vi "Teleop.vi"(10 "Match Info":T1={"Autonomous Elapsed Seconds"=0.0, "TeleOp Elapsed Seconds"=0.0, "Disabled Elapsed Seconds"=0.0, "Visited Autonomous"=FALSE, "Visited TeleOp"=FALSE, "Visited Disabled"=FALSE, "Autonomous Settings"={"Autonomous Style"=enum."Independent", "VI Refnum"=refnum}}, 11 "Call Context":T2) -> ()   [LabVIEW 2011]
doc: "This VI is called for each TeleOp packet received from the DS where the robot is not disabled. It is often used to read from the joysticks and update I/O or to update setpoints for timed control loops. It should complete and return within 20 milliseconds or it may miss DS packets."
uses:
  <vilib>/Rock Robotics/WPI/DriverStation/WPI_DriverStationDerivedRobotMode.ctl
  <vilib>/Rock Robotics/WPI/DriverStation/WPI_DriverStationMatch Info.ctl
  Robot Global Data.vi
panel:
  out "Position 4":dbl
  out "Position 3":dbl
  out "Shift Control":dbl=2.0 format="%.2f"
  in  "Left High":dbl=0.2
  in  "Right High":dbl=0.8
  in  "Left Mid":dbl=0.25
  in  "Right Mid":dbl=0.7
  in  "Shift Input 2":dbl
  in  "Left Low":dbl=0.8
  in  "Right Low":dbl=0.4
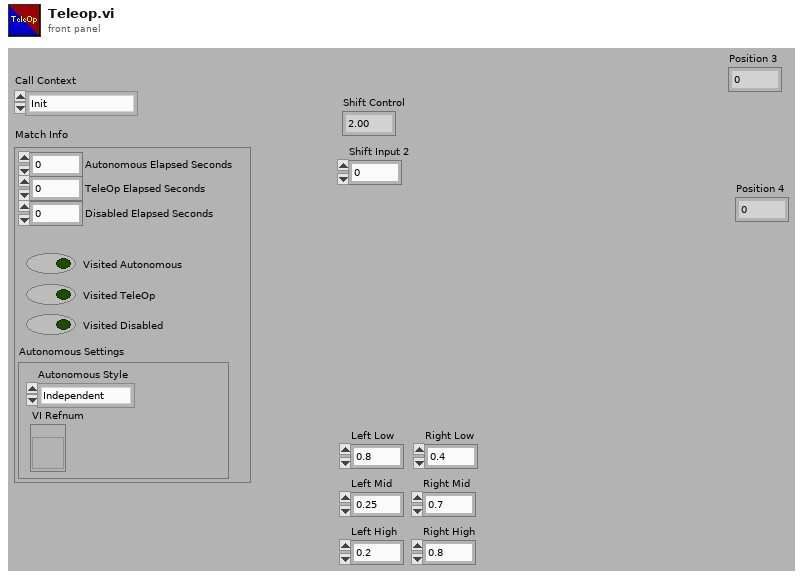
[diagram p1: front panel]
types:
  T1 = typedef "WPI_DriverStationMatch Info.ctl" = cluster{"Autonomous Elapsed Seconds":dbl, "TeleOp Elapsed Seconds":dbl, "Disabled Elapsed Seconds":dbl, "Visited Autonomous":bool, "Visited TeleOp":bool, "Visited Disabled":bool, "Autonomous Settings":cluster{"Autonomous Style":enum16{"Iterative", "Independent"}, "VI Refnum":refnum<vi>}}
  T2 = typedef "WPI_DriverStationDerivedRobotMode.ctl" = enum16{"Init", "Execute", "Stop"}
  T3 = typedef "WPI_JoystickDevRef.ctl" = cluster{"Device":T4}
  T4 = typedef "WPI_JoystickDeviceEnum.ctl" = enum16{"USB 1", "USB 2", "USB 3", "USB 4", "Kinect 1", "Kinect 2"}
  T5 = typedef "WPI_JoystickButtonState.ctl" = cluster{"Button 1":bool, "Button 2":bool, "Button 3":bool, "Button 4":bool, "Button 5":bool, "Button 6":bool, "Button 7":bool, "Button 8":bool, "Button 9":bool, "Button 10":bool, "Button 11":bool, "Button 12":bool}
  T6 = typedef "WPI_MotorControlDeviceRef.ctl" = cluster{"DeviceStatus":errorcluster, "Type":enum16{"PWM", "CAN"}, "PWM":cluster{"Digital Module":T7, "PWM Channel":T8, "DeadBand":T9}, "CAN":cluster{"Device Number":u8, "Control Mode":T10, "Semaphore":T11, "Max Vout":dbl}, "Invert":bool, "TransformRef":T12, "InvTransformRef":T12}
  T7 = typedef "FPGA_TypedefDigitalModule.ctl" = enum16{"Digital Module 1", "Digital Module 2"}
  T8 = typedef "FPGA_DIOPWMChannel.ctl" = enum8{"PWM 1", "PWM 2", "PWM 3", "PWM 4", "PWM 5", "PWM 6", "PWM 7", "PWM 8", "PWM 9", "PWM 10", "Invalid"}
  T9 = typedef "WPI_PWMDeadband.ctl" = cluster{"Name":string, "maxPositivePwm":i32, "minPositivePwm":i32, "centerPwm":i32, "maxNegativePwm":i32, "minNegativePwm":i32, "angularRange":u16}
  T10 = typedef "WPI_CANJaguar_ControlMode.ctl" = enum8{"Percent VBus", "Current", "Speed", "Position", "Voltage"}
  T11 = typedef "Semaphore RefNum" = refnum<k1>
  T12 = typedef "WPI_PWMTransform_ConPane.ctl" = refnum<vi>
  T13 = cluster{"axis 1 (x)":dbl, "axis 2 (y)":dbl, "axis 3 (throttle)":dbl, "axis 4":dbl, "axis 5":dbl, "axis 6":dbl}
  T14 = typedef "WPI_ServoDeviceRef.ctl" = cluster{"DeviceStatus":errorcluster, "Digital Module":T7, "PWM Channel":T8, "DeadBand":T9}
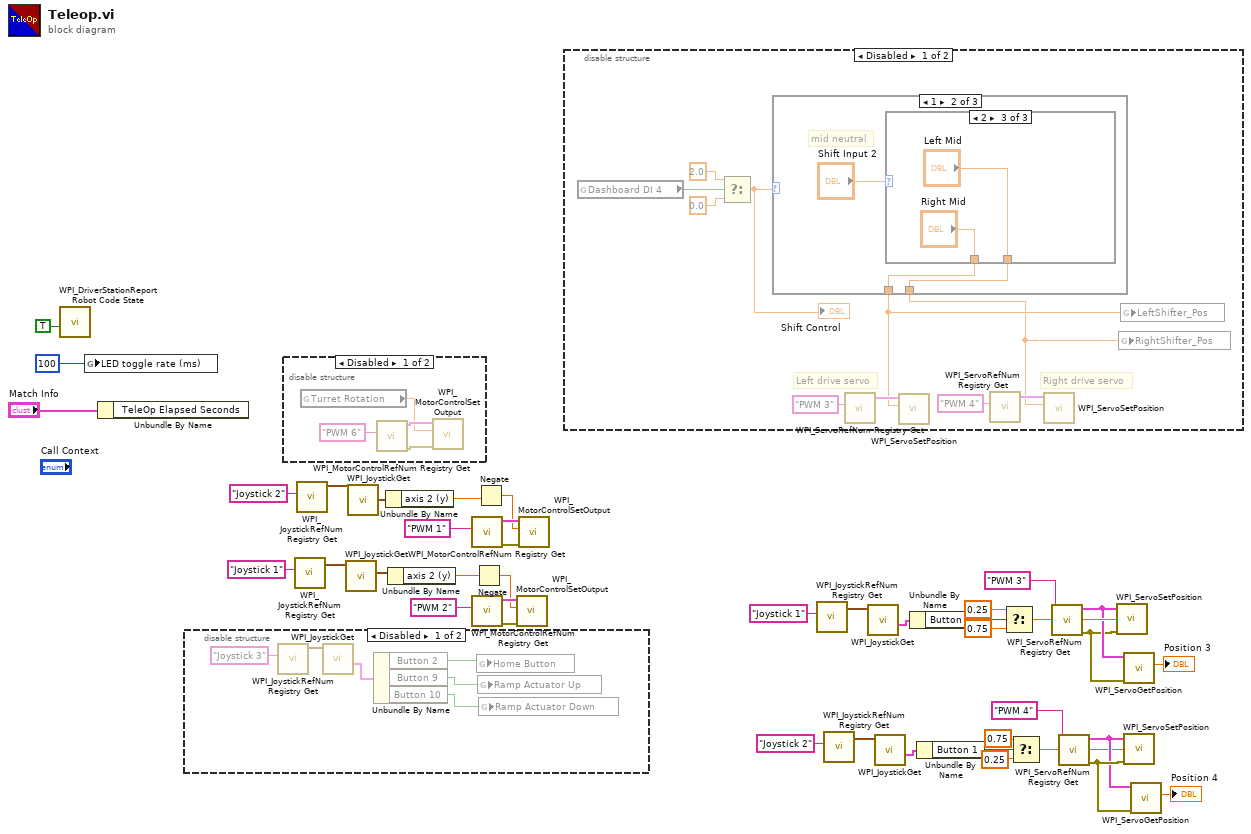
[diagram p0: block diagram]
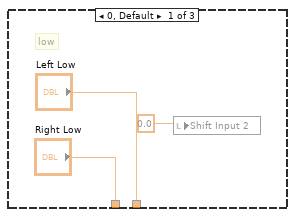
[diagram p4: hidden frame]
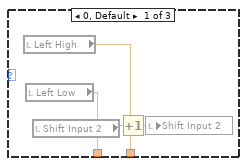
[diagram p5: hidden frame]
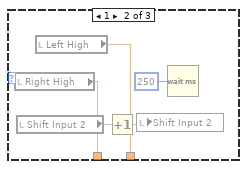
[diagram p6: hidden frame]
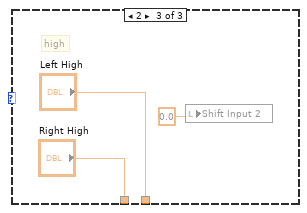
[diagram p7: hidden frame]
diagram:
  n1 = call <vilib>:"WPI_DriverStationReport Robot Code State.vi"("TeleOp"=TRUE ("Autonomous")) -> ()  [unwired: 10 in, 1 out]
  n2 = global write "Robot Global Data.vi" "LED toggle rate (ms)"(u32 100 ("LED ms toggle rate")) -> ()
  n3 = Unbundle By Name("Match Info") -> ()  [unwired: 1 out]
  n4 = disable-structure shown="Disabled" {
    frame Disabled {
      n5 = call <vilib>:"WPI_JoystickRefNum Registry Get.vi"("refnum name"="Joystick 3") -> ("JoystickDevRef"=w47:T3)  [unwired: 9 in, 1 out]
      n6 = call <vilib>:"WPI_JoystickGet.vi"("JoystickDevRef"=w47) -> ("Buttons"=w46:T5)  [unwired: 4 in, 2 out]
      n7 = Unbundle By Name(w46) -> ("Button 2"=w45:bool, "Button 9"=w43:bool, "Button 10"=w42:bool)
      n8 = global write "Robot Global Data.vi" "Home Button"(w45) -> ()
      n9 = global write "Robot Global Data.vi" "Ramp Actuator Up"(w43) -> ()
      n10 = global write "Robot Global Data.vi" "Ramp Actuator Down"(w42) -> ()
    }
    frame Enabled {
    }
  }
  n11 = disable-structure shown="Disabled" {
    frame Disabled {
      n12 = global read "Robot Global Data.vi" "Turret Rotation"() -> (w48:dbl)
      n13 = call <vilib>:"WPI_MotorControlRefNum Registry Get.vi"("refnum name"="PWM 6") -> ("error out"=w51:errorcluster, "MotorControlDevRef"=w50:T6)  [unwired: 9 in]
      n14 = call <vilib>:"WPI_MotorControlSetOutput.vi"("error in (no error)"=w51, "Output"=w48, "MotorControlDevRef"=w50) -> ()  [unwired: 7 in, 2 out]
    }
    frame Enabled {
    }
  }
  n15 = call <vilib>:"WPI_JoystickRefNum Registry Get.vi"("refnum name"="Joystick 1") -> ("JoystickDevRef"=w33:T3)  [unwired: 9 in, 1 out]
  n16 = call <vilib>:"WPI_JoystickRefNum Registry Get.vi"("refnum name"="Joystick 2") -> ("JoystickDevRef"=w36:T3)  [unwired: 9 in, 1 out]
  n17 = call <vilib>:"WPI_JoystickGet.vi"("JoystickDevRef"=w33) -> ("Axes"=w37:T13)  [unwired: 4 in, 2 out]
  n18 = call <vilib>:"WPI_JoystickGet.vi"("JoystickDevRef"=w36) -> ("Axes"=w38:T13)  [unwired: 4 in, 2 out]
  n19 = Unbundle By Name(w38) -> ("axis 2 (y)"=w26:dbl)
  n20 = Unbundle By Name(w37) -> ("axis 2 (y)"=w24:dbl)
  n21 = call <vilib>:"WPI_MotorControlRefNum Registry Get.vi"("refnum name"="PWM 1") -> ("error out"=w30:errorcluster, "MotorControlDevRef"=w29:T6)  [unwired: 9 in]
  n22 = call <vilib>:"WPI_MotorControlRefNum Registry Get.vi"("refnum name"="PWM 2") -> ("error out"=w32:errorcluster, "MotorControlDevRef"=w31:T6)  [unwired: 9 in]
  n23 = Negate(x=w24) -> (-x=w23:dbl)
  n24 = Negate(x=w26) -> (-x=w25:dbl)
  n25 = call <vilib>:"WPI_MotorControlSetOutput.vi"("error in (no error)"=w32, "Output"=w23, "MotorControlDevRef"=w31) -> ()  [unwired: 7 in, 2 out]
  n26 = call <vilib>:"WPI_MotorControlSetOutput.vi"("error in (no error)"=w30, "Output"=w25, "MotorControlDevRef"=w29) -> ()  [unwired: 7 in, 2 out]
  n27 = disable-structure shown="Disabled" {
    frame Disabled {
      # "Right drive servo"
      # "Left drive servo"
      n28 = global read "Robot Global Data.vi" "Dashboard DI 4"() -> (w54:bool)
      n29 = Select(t=2.0, s=w54, f=0.0) -> (s? t:f=w56:dbl)
      "Shift Control" <- w56
      n30 = case shown="1" w56 {
        tunnel: ["Left Low" w66 "Left High"] -> w52
        tunnel: ["Right Low" w65 "Right High"] -> w53
        frame 0, Default {
          # "low"
          n31 = local write "Shift Input 2"(0.0 ("Input 2")) -> ()
        }
        frame 1 {
          # "mid neutral"
          n32 = case shown="2" "Shift Input 2" {
            tunnel: [w71 w72 "Left Mid"] -> w66
            tunnel: [w70 w73 "Right Mid"] -> w65
            frame 0, Default {
              n33 = local read "Left High"() -> (w71:dbl)
              n34 = local read "Left Low"() -> (w70:dbl)
              n35 = local read "Shift Input 2"() -> (w69:dbl)
              n36 = Increment(x=w69) -> (x+1=w68:dbl)
              n37 = local write "Shift Input 2"(w68) -> ()
            }
            frame 1 {
              n38 = local read "Right High"() -> (w73:dbl)
              n39 = local read "Shift Input 2"() -> (w75:dbl)
              n40 = local read "Left High"() -> (w72:dbl)
              n41 = Increment(x=w75) -> (x+1=w74:dbl)
              n42 = local write "Shift Input 2"(w74) -> ()
              n43 = Wait (ms)(milliseconds to wait=u32 250) -> ()  [unwired: 1 out]
            }
            frame 2 {
            }
          }
        }
        frame 2 {
          # "high"
          n44 = local write "Shift Input 2"(0.0 ("Input 2")) -> ()
        }
      }
      n45 = call <vilib>:"WPI_ServoRefNum Registry Get.vi"("refnum name"="PWM 3") -> ("ServoDeviceRef"=w61:T14)  [unwired: 1 in, 9 out]
      n46 = call <vilib>:"WPI_ServoSetPosition.vi"("Position"=w53, "ServoDeviceRef"=w61) -> ()  [unwired: 1 in, 9 out]
      n47 = call <vilib>:"WPI_ServoRefNum Registry Get.vi"("refnum name"="PWM 4") -> ("ServoDeviceRef"=w57:T14)  [unwired: 1 in, 9 out]
      n48 = call <vilib>:"WPI_ServoSetPosition.vi"("Position"=w52, "ServoDeviceRef"=w57) -> ()  [unwired: 1 in, 9 out]
      n49 = global write "Robot Global Data.vi" "RightShifter_Pos"(w52) -> ()
      n50 = global write "Robot Global Data.vi" "LeftShifter_Pos"(w53) -> ()
    }
    frame Enabled {
    }
  }
  n51 = call <vilib>:"WPI_JoystickRefNum Registry Get.vi"("refnum name"="Joystick 1") -> ("JoystickDevRef"=w22:T3)  [unwired: 9 in, 1 out]
  n52 = call <vilib>:"WPI_JoystickRefNum Registry Get.vi"("refnum name"="Joystick 2") -> ("JoystickDevRef"=w1:T3)  [unwired: 9 in, 1 out]
  n53 = call <vilib>:"WPI_JoystickGet.vi"("JoystickDevRef"=w22) -> ("Buttons"=w20:T5)  [unwired: 4 in, 2 out]
  n54 = call <vilib>:"WPI_JoystickGet.vi"("JoystickDevRef"=w1) -> ("Buttons"=w3:T5)  [unwired: 4 in, 2 out]
  n55 = Unbundle By Name(w20) -> ("Button 1"=w19:bool)
  n56 = Unbundle By Name(w3) -> ("Button 1"=w4:bool)
  n57 = Select(t=0.25, s=w19, f=0.75) -> (s? t:f=w16:dbl)
  n58 = Select(t=0.75, s=w4, f=0.25) -> (s? t:f=w7:dbl)
  n59 = call <vilib>:"WPI_ServoRefNum Registry Get.vi"("refnum name"="PWM 3") -> ("error out"=w13:errorcluster, "ServoDeviceRef"=w14:T14)  [unwired: 9 in]
  n60 = call <vilib>:"WPI_ServoRefNum Registry Get.vi"("refnum name"="PWM 4") -> ("error out"=w10:errorcluster, "ServoDeviceRef"=w9:T14)  [unwired: 9 in]
  n61 = call <vilib>:"WPI_ServoSetPosition.vi"("error in (no error)"=w13, "Position"=w16, "ServoDeviceRef"=w14) -> ()  [unwired: 7 in, 2 out]
  n62 = call <vilib>:"WPI_ServoGetPosition.vi"("error in (no error)"=w13, "ServoDeviceRef"=w14) -> ("Position"=→"Position 3":dbl)  [unwired: 7 in, 2 out]
  n63 = call <vilib>:"WPI_ServoSetPosition.vi"("error in (no error)"=w10, "Position"=w7, "ServoDeviceRef"=w9) -> ()  [unwired: 7 in, 2 out]
  n64 = call <vilib>:"WPI_ServoGetPosition.vi"("error in (no error)"=w10, "ServoDeviceRef"=w9) -> ("Position"=→"Position 4":dbl)  [unwired: 7 in, 2 out]
